vi "Channels.Format.vi"(8 "error in (no error)":errorcluster, 11 "Channels":string[](array[string])) -> (0 "error out":errorcluster, 2 "Channels":T1[](array[typedef]), 3 "Channels (no blanks)":T1[](array[typedef]))   [LabVIEW 2015, in "Single Station Execution.lvlib"]
uses:
  Single Station Execution.lvlib
  Types/Channel.Properties.ctl
  NationalInstruments.VeriStand
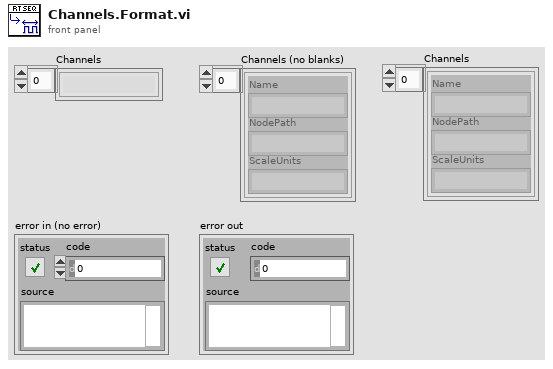
[diagram p1: front panel]
types:
  T1 = typedef "Single Station Execution.lvlib/Channel.Properties.ctl" = cluster{"Name":string, "NodePath":string, "ScaleUnits":string}
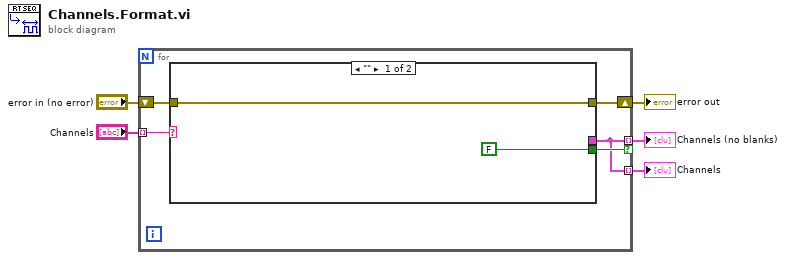
[diagram p0: block diagram]
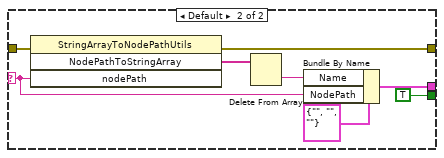
[diagram p2: hidden frame]
diagram:
  n1 = for {
    tunnel: "Channels" -> [w8] mode=indexing
    tunnel: [w6] -> w3 mode=indexing if=w7
    shift-right: [w9] -> w4
    shift-left: "error in (no error)" -> [w10]
    tunnel: [w6] -> w1 mode=indexing
    n2 = case shown="\"\"" w8 {
      selector: w8 -> [_ w14]
      tunnel: [_ w17] -> w6
      tunnel: w10 -> [w12 w16]
      tunnel: [w12 w15] -> w9
      tunnel: [FALSE TRUE] -> w7
      frame "" {
      }
      frame Default {
        n3 = invoke class="StringArrayToNodePathUtils" method="NodePathToStringArray"(error in=w16, "nodePath"=w14) -> (error out=w15:errorcluster, "NodePathToStringArray"=w20:string[])  [unwired: 2 in, 2 out]
        n4 = Delete From Array(array=w20) -> (deleted portion=w18:string)  [unwired: 2 in, 1 out]
        n5 = Bundle By Name(cluster=T1 {"Name"="", "NodePath"="", "ScaleUnits"=""} ("Channel"), "Name"=w18, "NodePath"=w14) -> (w17:T1)
      }
    }
  }
  "error out" <- w4
  "Channels (no blanks)" <- w3
  "Channels" <- w1
